vi "Periodic String Speed Check.vi"(7 "Reset?":bool, 8 "Settings":T1={"threashold(#/s)"=1.0, "Check Peroid(s)"=1.0}, 10 "Seconds Since 1Jan1904":timestamp, 11 "Element":string) -> (0 "Over Threashold?":bool, 1 "Peroid?":bool, 2 "Timestamp":timestamp, 3 "X+1":i64)   [LabVIEW 2017]
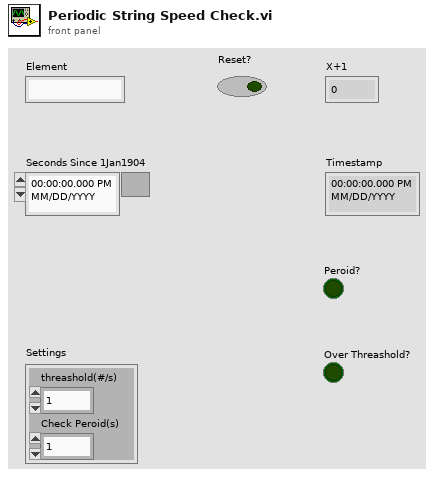
[diagram p1: front panel]
types:
  T1 = cluster{"threashold(#/s)":dbl, "Check Peroid(s)":dbl}
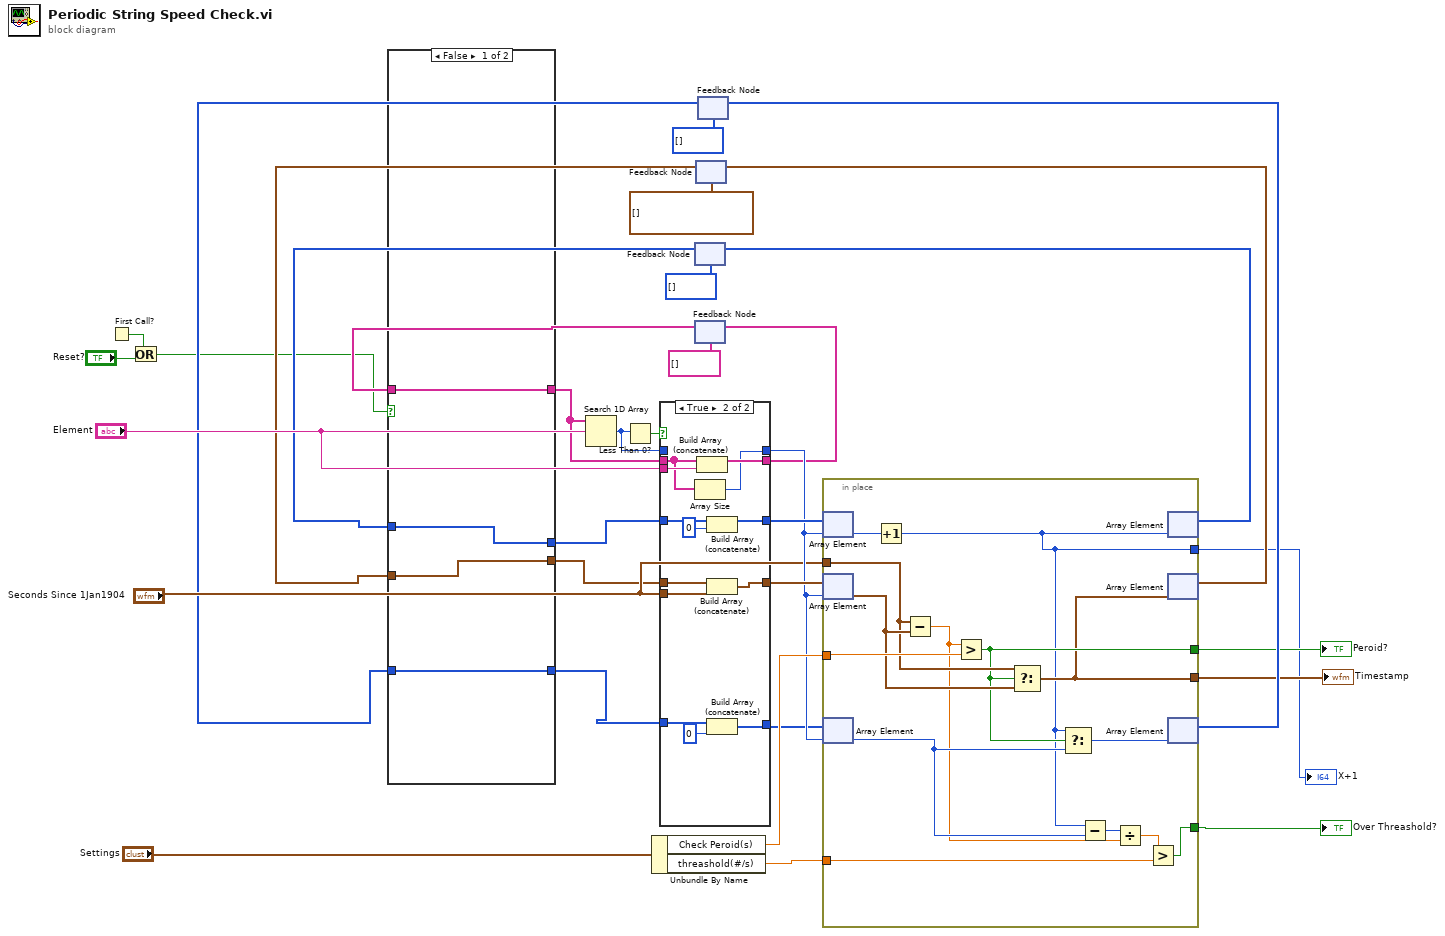
[diagram p0: block diagram]
diagram:
  n1 = First Call?() -> (First Call?: T/F=w3:bool)
  n2 = Or(x=w3, y="Reset?") -> (x .or. y?=w1:bool)
  n3 = Unbundle By Name("Settings") -> ("Check Peroid(s)"=w27:dbl, "threashold(#/s)"=w19:dbl)
  n4 = feedback #1(i64[] [] ("Input String 2")) -> (w9:i64[])
  n5 = feedback #2(string[] [] ("Input String 2")) -> (w10:string[])
  n6 = feedback #3(timestamp[] [] ("Input String 2")) -> (w7:timestamp[])
  n7 = feedback #4(i64[] [] ("Input String 2")) -> (w5:i64[])
  n8 = case shown="False" w1 {
    tunnel: [w38 _] -> w11
    tunnel: w10 -> [w38 _]
    tunnel: [w37 _] -> w8
    tunnel: w9 -> [w37 _]
    tunnel: [w36 _] -> w6
    tunnel: w7 -> [w36 _]
    tunnel: w5 -> [w35 _]
    tunnel: [w35 _] -> w4
    frame False {
    }
    frame True {
    }
  }
  n9 = Search 1D Array(1D array=w11, element="Element") -> (index of element=w31:i32)  [unwired: 1 in]
  n10 = Less Than 0?(x=w31) -> (x < 0?=w32:bool)
  n11 = case shown="True" w32 {
    tunnel: w11 -> [w43 w54]
    tunnel: "Element" -> [_ w56]
    tunnel: [w43 w55] -> w23
    tunnel: w31 -> [w42 _]
    tunnel: [w42 w53] -> w25
    tunnel: w8 -> [w41 w52]
    tunnel: [w41 w50] -> w30
    tunnel: w6 -> [w40 w49]
    tunnel: "Seconds Since 1Jan1904" -> [_ w48]
    tunnel: [w40 w47] -> w28
    tunnel: w4 -> [w39 w46]
    tunnel: [w39 w44] -> w24
    frame False {
    }
    frame True {
      n12 = Array Size(array=w54) -> (size(s)=w53:i32)
      n13 = Build Array (concatenate)(w54, w56) -> (w55:string[])
      n14 = Build Array (concatenate)(w52, i64 0 ("64bit integer")) -> (w50:i64[])
      n15 = Build Array (concatenate)(w49, w48) -> (w47:timestamp[])
      n16 = Build Array (concatenate)(w46, i64 0 ("64bit integer")) -> (w44:i64[])
    }
  }
  n17 = feedback-in #2(w23) -> ()
  n18 = in-place {
    in-place-border: "Seconds Since 1Jan1904" -> [w67]
    in-place-border: w27 -> [w69]
    in-place-border: [w66] -> w16
    in-place-border: [w64] -> w14
    in-place-border: w19 -> [w59]
    in-place-border: [w58] -> w15
    in-place-border: [w57] -> w12
    n19 = in-place-array #5(w30, w25) -> (w70:i64)
    n20 = in-place-array #6(w28, w25) -> (w68:timestamp)
    n21 = in-place-array #7(w24, w25) -> (w61:i64)
    n22 = Increment(x=w70) -> (x+1=w57:i64)
    n23 = Subtract(x=w67, y=w68) -> (x-y=w60:dbl)
    n24 = Greater?(x=w60, y=w69) -> (0:w66:bool)
    n25 = Select(t=w67, s=w66, f=w68) -> (s? t:f=w64:timestamp)
    n26 = Select(t=w57, s=w66, f=w61) -> (s? t:f=w65:i64)
    n27 = Subtract(x=w57, y=w61) -> (x-y=w62:i64)
    n28 = Divide(x=w62, y=w60) -> (x/y=w63:dbl)
    n29 = Greater?(x=w63, y=w59) -> (0:w58:bool)
    n30 = in-place-array #5(w57) -> (w22:i64[])  [unwired: 1 out]
    n31 = in-place-array #6(w64) -> (w21:timestamp[])  [unwired: 1 out]
    n32 = in-place-array #7(w65) -> (w20:i64[])  [unwired: 1 out]
  }
  "Peroid?" <- w16
  "Over Threashold?" <- w15
  "Timestamp" <- w14
  "X+1" <- w12
  n33 = feedback-in #1(w22) -> ()
  n34 = feedback-in #3(w21) -> ()
  n35 = feedback-in #4(w20) -> ()
